vi "Pixie4SaveDSPParToFile.vi"(1 "DSP parameters file (.set file in folder \"Configuration\")":path=path "D:/dsp files") -> (0 "Return value":i32)   [LabVIEW 2016]
uses:
  Drivers/Pixie4DLL.dll
panel:
  in  "OK Button":bool
  # "0  - saving DSP parameters to file successful\n-1  - failed to save DSP parameters to file"
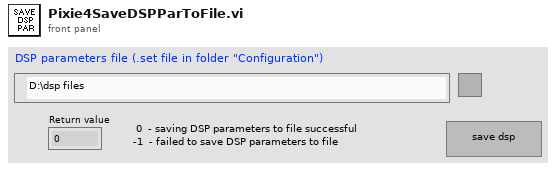
[diagram p1: front panel]
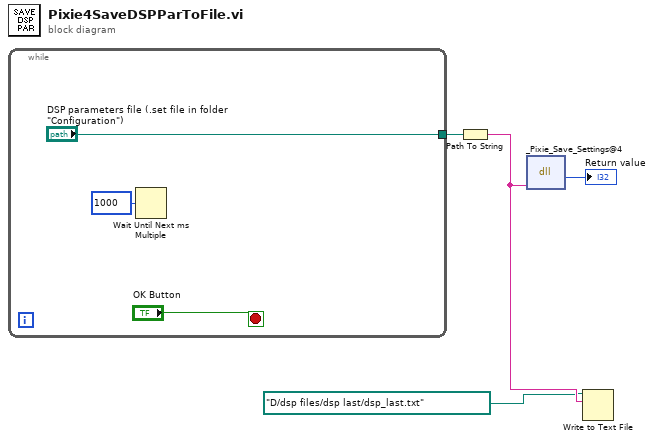
[diagram p0: block diagram]
diagram:
  n1 = while {
    tunnel: ["DSP parameters file (.set file in folder \"Configuration\")"] -> w4
    stop <- "OK Button" stop-if-true
    n2 = Wait Until Next ms Multiple(millisecond multiple=u32 1000) -> ()  [unwired: 1 out]
  }
  n3 = Path To String(path=w4) -> (string=w2:string)
  n4 = dll-call lib="D:/Users/wymanm/Desktop/DAQuiri - 2017a/PRIME DAQ 2017a/Drivers/Pixie4DLL.dll" fn="_Pixie_Save_Settings@4"("DSPSettingsFile"=w2) -> ("return type"=→"Return value":i32)  [unwired: 4 in, 2 out]
  n5 = Write to Text File(file (use dialog)=path "D:/dsp files/dsp last/dsp_last.txt", text=w2) -> ()  [unwired: 2 in, 3 out]
